vi "Get Size of Data from TD - Benchmark Map Collection of Fixed-size Key and Value (I32,I32) - Should Perform in O(1)+O(1).vi"() -> ()   [LabVIEW 2017, in "Composition.Tests.lvlib"]
uses:
  Composition.Tests.lvlib
  <vilib>/addons/_JKI Toolkits/Caraya/classes/Assert/Assert Less_Variant.vi
  Composition/Composition.lvlib
  <vilib>/addons/_JKI Toolkits/Caraya/classes/Test/Test.lvclass
  <vilib>/addons/_JKI Toolkits/Caraya/classes/Assert/Assert.lvclass
panel:
  out "error out":errorcluster
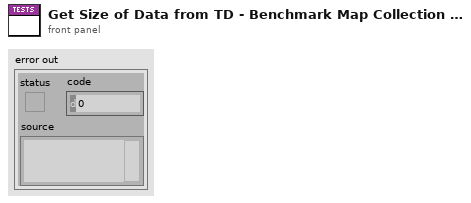
[diagram p1: front panel]
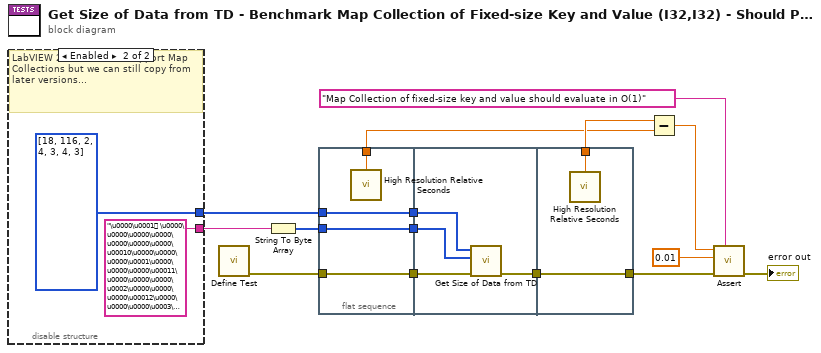
[diagram p0: block diagram]
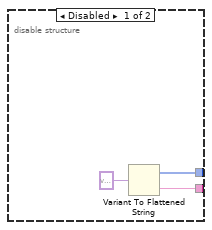
[diagram p2: hidden frame]
diagram:
  n1 = disable-structure shown="Enabled" {
    disable-tunnel: [w18 "\u0000\u0001 \u0000\u0000\u0000\u0000\u0000\u0000\u0000\u00010\u0000\u0000\u0000\u0001\u0000\u0000\u0000\u00011\u0000\u0000\u0000\u0002\u0000\u0000\u0000\u00012\u0000\u0000\u0000\u0003\u0000\u0000\u0000\u00013\u0000\u0000\u0000\u0004\u0000\u0000\u0000\u00014\u0000\u0000\u0000\u0005\u0000\u0000\u0000\u00015\u0000\u0000\u0000\u0006\u0000\u0000\u0000\u00016\u0000\u0000\u0000\u0007\u0000\u0000\u0000\u00017\u0000\u0000\u0000\b\u0000\u0000\u0000\u00018\u0000\u0000\u0000\t\u0000\u0000\u0000\u00019\u0000\u0000\u0000\n\u0000\u0000\u0000\u000210\u0000\u0000\u0000\u000b\u0000\u0000\u0000\u000211\u0000\u0000\u0000\f\u0000\u0000\u0000\u000212\u0000\u0000\u0000\r\u0000\u0000\u0000\u000213\u0000\u0000\u0000\u000e\u0000\u0000\u0000\u000214\u0000\u0000\u0000\u000f\u0000\u0000\u0000\u000215\u0000\u0000\u0000\u0010\u0000\u0000\u0000\u000216\u0000\u0000\u0000\u0011\u0000\u0000\u0000\u000217\u0000\u0000\u0000\u0012\u0000\u0000\u0000\u000218\u0000\u0000\u0000\u0013\u0000\u0000\u0000\u000219\u0000\u0000\u0000\u0014\u0000\u0000\u0000\u000220\u0000\u0000\u0000\u0015\u0000\u0000\u0000\u000221\u0000\u0000\u0000\u0016\u0000\u0000\u0000\u000222\u0000\u0000\u0000\u0017\u0000\u0000\u0000\u000223\u0000\u0000\u0000\u0018\u0000\u0000\u0000\u000224\u0000\u0000\u0000\u0019\u0000\u0000\u0000\u000225\u0000\u0000\u0000\u001a\u0000\u0000\u0000\u000226\u0000\u0000\u0000\u001b\u0000\u0000\u0000\u000227\u0000\u0000\u0000\u001c\u0000\u0000\u0000\u000228\u0000\u0000\u0000\u001d\u0000\u0000\u0000\u000229\u0000\u0000\u0000\u001e\u0000\u0000\u0000\u000230\u0000\u0000\u0000\u001f\u0000\u0000\u0000\u000231\u0000\u0000\u0000 \u0000\u0000\u0000\u000232\u0000\u0000\u0000!\u0000\u0000\u0000\u000233\u0000\u0000\u0000\"\u0000\u0000\u0000\u000234\u0000\u0000\u0000#\u0000\u0000\u0000\u000235\u0000\u0000\u0000$\u0000\u0000\u0000\u000236\u0000\u0000\u0000%\u0000\u0000\u0000\u000237\u0000\u0000\u0000&\u0000\u0000\u0000\u000238\u0000\u0000\u0000'\u0000\u0000\u0000\u000239\u0000\u0000\u0000(\u0000\u0000\u0000\u000240\u0000\u0000\u0000)\u0000\u0000\u0000\u000241\u0000\u0000\u0000*\u0000\u0000\u0000\u000242\u0000\u0000\u0000+\u0000\u0000\u0000\u000243\u0000\u0000\u0000,\u0000\u0000\u0000\u000244\u0000\u0000\u0000-\u0000\u0000\u0000\u000245\u0000\u0000\u0000.\u0000\u0000\u0000\u000246\u0000\u0000\u0000/\u0000\u0000\u0000\u000247\u0000\u0000\u00000\u0000\u0000\u0000\u000248\u0000\u0000\u00001\u0000\u0000\u0000\u000249\u0000\u0000\u00002\u0000\u0000\u0000\u000250\u0000\u0000\u00003\u0000\u0000\u0000\u000251\u0000\u0000\u00004\u0000\u0000\u0000\u000252\u0000\u0000\u00005\u0000\u0000\u0000\u000253\u0000\u0000\u00006\u0000\u0000\u0000\u000254\u0000\u0000\u00007\u0000\u0000\u0000\u000255\u0000\u0000\u00008\u0000\u0000\u0000\u000256\u0000\u0000\u00009\u0000\u0000\u0000\u000257\u0000\u0000\u0000:\u0000\u0000\u0000\u000258\u0000\u0000\u0000;\u0000\u0000\u0000\u000259\u0000\u0000\u0000<\u0000\u0000..." ("data string")] -> w1
    disable-tunnel: [w16 i16[] [18, 116, 2, 4, 3, 4, 3] ("Type Descriptor")] -> w2
    frame Disabled {
      n2 = Variant To Flattened String(Variant=variant) -> (data string=w18:string, 1:w16:i16[])
    }
    frame Enabled {
      # "LabVIEW 2017 does not support Map Collections but we can still copy from later versions..."
    }
  }
  n3 = call <vilib>:"Define Test.vi"() -> ("error out"=w14:errorcluster)  [unwired: 11 in]
  n4 = String To Byte Array(string=w1) -> (unsigned byte array=w15:u8[])
  n5 = flat-sequence {
    tunnel: w14 -> [w22]
    tunnel: w15 -> [w23]
    tunnel: w2 -> [w24]
    tunnel: [w24] -> w13
    tunnel: [w23] -> w12
    tunnel: [w22] -> w11
    tunnel: [w21] -> w9
    tunnel: w13 -> [w28]
    tunnel: w12 -> [w27]
    tunnel: w11 -> [w26]
    tunnel: [w25] -> w8
    tunnel: [w30] -> w10
    tunnel: [w29] -> w7
    tunnel: w8 -> [w29]
    frame #0 {
      n6 = call <vilib>:"High Resolution Relative Seconds.vi"() -> ("relative seconds"=w21:dbl)
    }
    frame #1 {
      n7 = call "Get Size of Data from TD.vi"("error in (no error)"=w26, "Data String"=w27, "Type Descriptor"=w28) -> ("error out"=w25:errorcluster)  [unwired: 7 in, 1 out]
    }
    frame #2 {
      n8 = call <vilib>:"High Resolution Relative Seconds.vi"() -> ("relative seconds"=w30:dbl)
    }
  }
  n9 = Subtract(x=w10, y=w9) -> (x-y=w6:dbl)
  n10 = call-poly <vilib>:"Assert.vi"("Label"="Map Collection of fixed-size key and value should evaluate in O(1)", "error in (no error)"=w7, "Y"=0.01 ("x-y"), "X"=w6) -> ("error out"=→"error out":errorcluster)  [unwired: 7 in]
